vi "State Machine Example.vi"() -> ()   [LabVIEW 2013]
uses:
  <vilib>/Utility/file.llb/Read From Spreadsheet File (string).vi
panel:
  out "Maze":string[][](table)
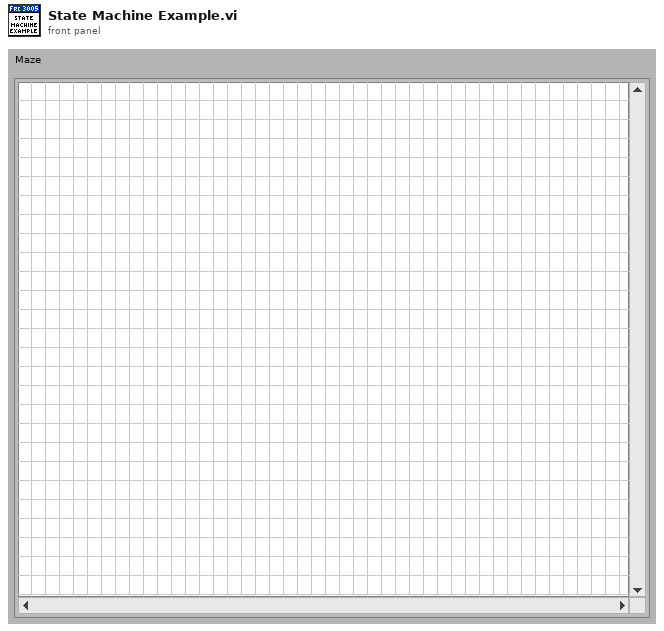
[diagram p1: front panel]
types:
  T1 = cluster{"String":string, "Numeric":dbl, "Array":bool[], "Enum":enum16{"Init", ""}}
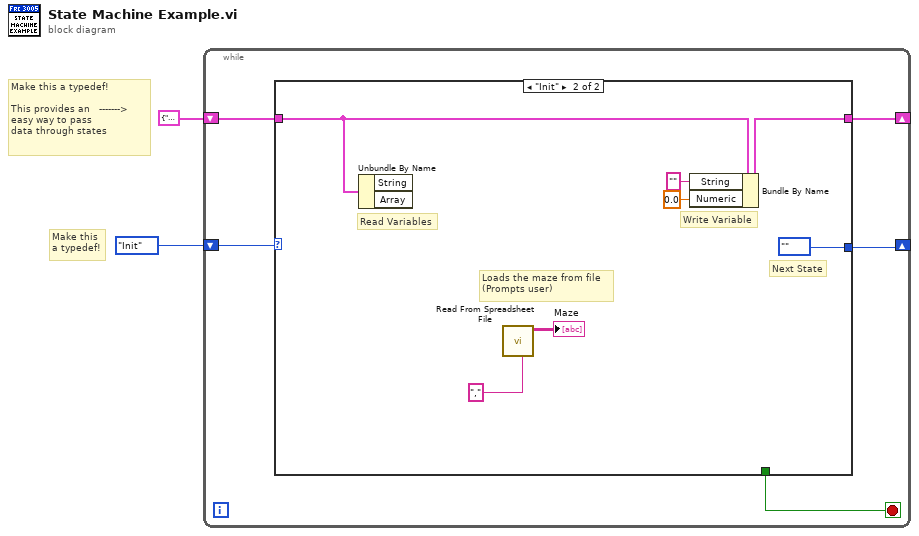
[diagram p0: block diagram]
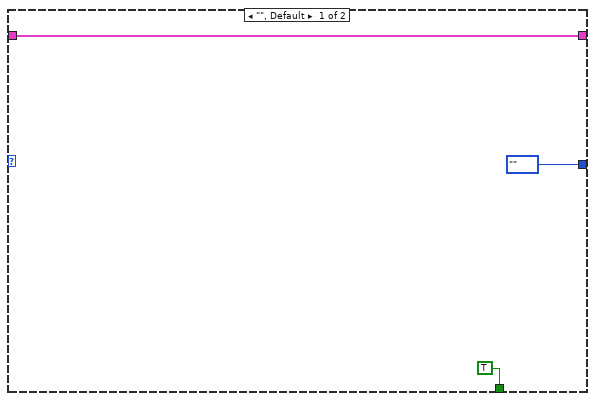
[diagram p2: hidden frame]
diagram:
  # "Make this\na typedef!"
  # "Make this a typedef!\n\nThis provides an   ------->\neasy way to pass\ndata through states"
  n1 = while {
    shift-right: [w6] -> _
    shift-left: enum16{"Init", ""}."Init" -> [w7]
    shift-right: [w3] -> _
    shift-left: T1 {"String"="", "Numeric"=0.0, "Array"=[], "Enum"=enum."Init"} ("Cluster") -> [w4]
    stop <- w5 stop-if-true
    n2 = case shown="\"Init\"" w7 {
      tunnel: [enum16{"Init", ""}."" enum16{"Init", ""}.""] -> w6
      tunnel: [TRUE _] -> w5
      tunnel: [w8 w14] -> w3
      tunnel: w4 -> [w8 w13]
      frame "", Default {
      }
      frame "Init" {
        # "Next State"
        # "Write Variable"
        # "Read Variables"
        # "Loads the maze from file\n(Prompts user)"
        n3 = Unbundle By Name(w13) -> ()  [unwired: 2 out]
        n4 = call-poly <vilib>:"Read From Spreadsheet File.vi"("delimiter (\\t)"="," ("delimiter (\\t)")) -> ("all rows"=→"Maze":string[][])  [unwired: 6 in, 4 out]
        n5 = Bundle By Name(cluster=w13, "String"="", "Numeric"=0.0) -> (w14:T1)
      }
    }
  }
